vi "CMI Sync V3 Set Channel 1 Division Factor by Desired Freq.vi"(8 "error in":errorcluster, 9 "explicit ref freq [Hz] (0: auto estimate)":dbl, 10 "target output freq [Hz]":dbl=1000.0, 11 "session in":T1={"VISA"="", "baud rate [bd/s]"=115200, "source"=enum."Auto", "hv range"=enum."1kV", "fsrc is fixed"=FALSE, "fsrc [Hz]"=10000000.0, "freq integ [s]"=1.0, "freq filter"=5, "trig level"=enum."TTL 5V", "chn1 mode"=enum."Source divider", "chn1 level"=enum."Positive 5V", "chn2 mode"=enum."Source divider", "chn2 level"=enum."Positive 5V", "chn2 div"=1, "chn3 mode"=enum."Chn 1 Active", "chn3 level"=enum."Positive 5V", "chn1 div entry"=enum."Calculate nearest divisor from measured fx", "chn1 dev limit [%]"=1.0, "chn1 check dev"=FALSE} {"chn2 div" min=1 max=100000000 step=1; "fsrc [Hz]" format="%_8p"}) -> (0 "error out":errorcluster, 1 "divisor":i32, 2 "output freq [Hz]":dbl, 3 "session out":T1={"VISA"="", "baud rate [bd/s]"=115200, "source"=enum."Auto", "hv range"=enum."1kV", "fsrc is fixed"=FALSE, "fsrc [Hz]"=10000000.0, "freq integ [s]"=1.0, "freq filter"=5, "trig level"=enum."TTL 5V", "chn1 mode"=enum."Source divider", "chn1 level"=enum."Positive 5V", "chn2 mode"=enum."Source divider", "chn2 level"=enum."Positive 5V", "chn2 div"=1, "chn3 mode"=enum."Chn 1 Active", "chn3 level"=enum."Positive 5V", "chn1 div entry"=enum."Calculate nearest divisor from measured fx", "chn1 dev limit [%]"=1.0, "chn1 check dev"=FALSE} {"chn2 div" min=1 max=100000000 step=1; "fsrc [Hz]" format="%_8p"})   [LabVIEW 2020, in "AWG.lvlib" / "CMI Sync Unit V3.lvlib"]
doc: "Sets nearest divisor for channel 1 in direct division mode by entering desired frequency and measured source frequency. Returns actual divisor and output frequency."
uses:
  CMI Sync Unit V3.lvlib
  CMI Sync V3 session.ctl
  CMI Sync V3 Reference Clock Source.ctl
  CMI Sync V3 HV input Range.ctl
  CMI Sync V3 Trigger Input Level.ctl
  CMI Sync V3 Channel 1 Mode.ctl
  CMI Sync V3 Channel Output Levels.ctl
  CMI Sync V3 Channel 2 Mode.ctl
  CMI Sync V3 Channel 3 Mode.ctl
  CMI Sync V3 Channel 1 Divisor Entry Mode.ctl
  <vilib>/Utility/error.llb/Error Cluster From Error Code.vi
  <vilib>/ErrorRing/Error Ring.xnode
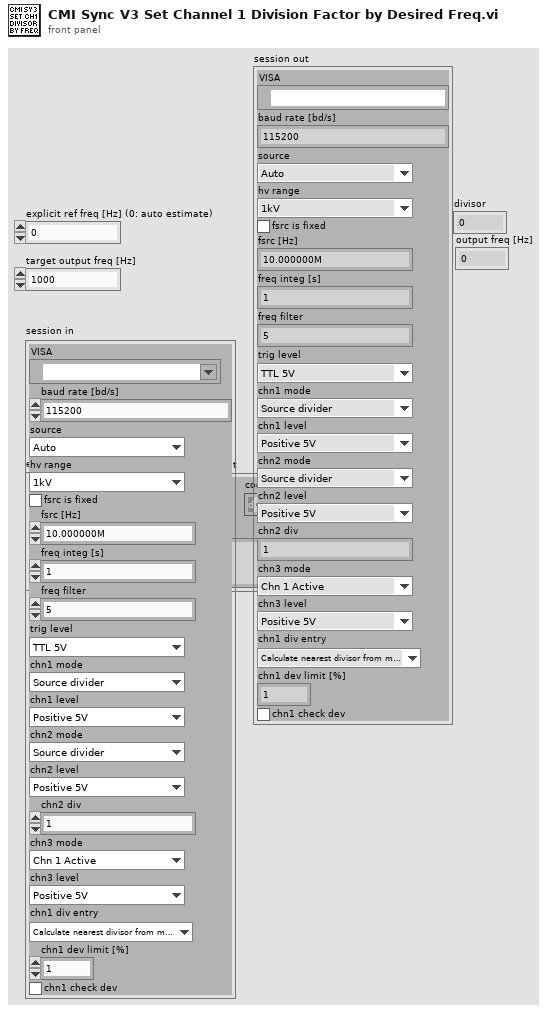
[diagram p1: front panel]
types:
  T1 = typedef "AWG.lvlib/CMI Sync Unit V3.lvlib/CMI Sync V3 session.ctl" = cluster{"VISA":refnum<visa-resource-name>, "baud rate [bd/s]":i32, "source":T2, "hv range":T3, "fsrc is fixed":bool, "fsrc [Hz]":dbl, "freq integ [s]":dbl, "freq filter":i32, "trig level":T4, "chn1 mode":T5, "chn1 level":T6, "chn2 mode":T7, "chn2 level":T6, "chn2 div":i32, "chn3 mode":T8, "chn3 level":T6, "chn1 div entry":T9, "chn1 dev limit [%]":dbl, "chn1 check dev":bool}
  T2 = typedef "AWG.lvlib/CMI Sync Unit V3.lvlib/CMI Sync V3 Reference Clock Source.ctl" = enum16{"Auto", "Internal", "Logic", "Sine", "HV"}
  T3 = typedef "AWG.lvlib/CMI Sync Unit V3.lvlib/CMI Sync V3 HV input Range.ctl" = enum16{"10V", "60V", "250V", "1kV"}
  T4 = typedef "AWG.lvlib/CMI Sync Unit V3.lvlib/CMI Sync V3 Trigger Input Level.ctl" = enum16{"LVCMOS 3V3", "TTL 5V"}
  T5 = typedef "AWG.lvlib/CMI Sync Unit V3.lvlib/CMI Sync V3 Channel 1 Mode.ctl" = enum16{"Source divider", "DDS absolute", "DDS ratio", "DDS ratio M/N"}
  T6 = typedef "AWG.lvlib/CMI Sync Unit V3.lvlib/CMI Sync V3 Channel Output Levels.ctl" = enum16{"Positive 3V3", "Negative 3V3", "Positive 5V", "Negative 5V"}
  T7 = typedef "AWG.lvlib/CMI Sync Unit V3.lvlib/CMI Sync V3 Channel 2 Mode.ctl" = enum16{"Source divider", "Chn 1 divide"}
  T8 = typedef "AWG.lvlib/CMI Sync Unit V3.lvlib/CMI Sync V3 Channel 3 Mode.ctl" = enum16{"Chn 1 Active", "Chn 2 Active", "Chn 1 Trigger", "Chn 2 Trigger", "Gate", "PPS", "10MHz"}
  T9 = typedef "AWG.lvlib/CMI Sync Unit V3.lvlib/CMI Sync V3 Channel 1 Divisor Entry Mode.ctl" = enum16{"Set divisor directly", "Calculate nearest divisor from measured fx"}
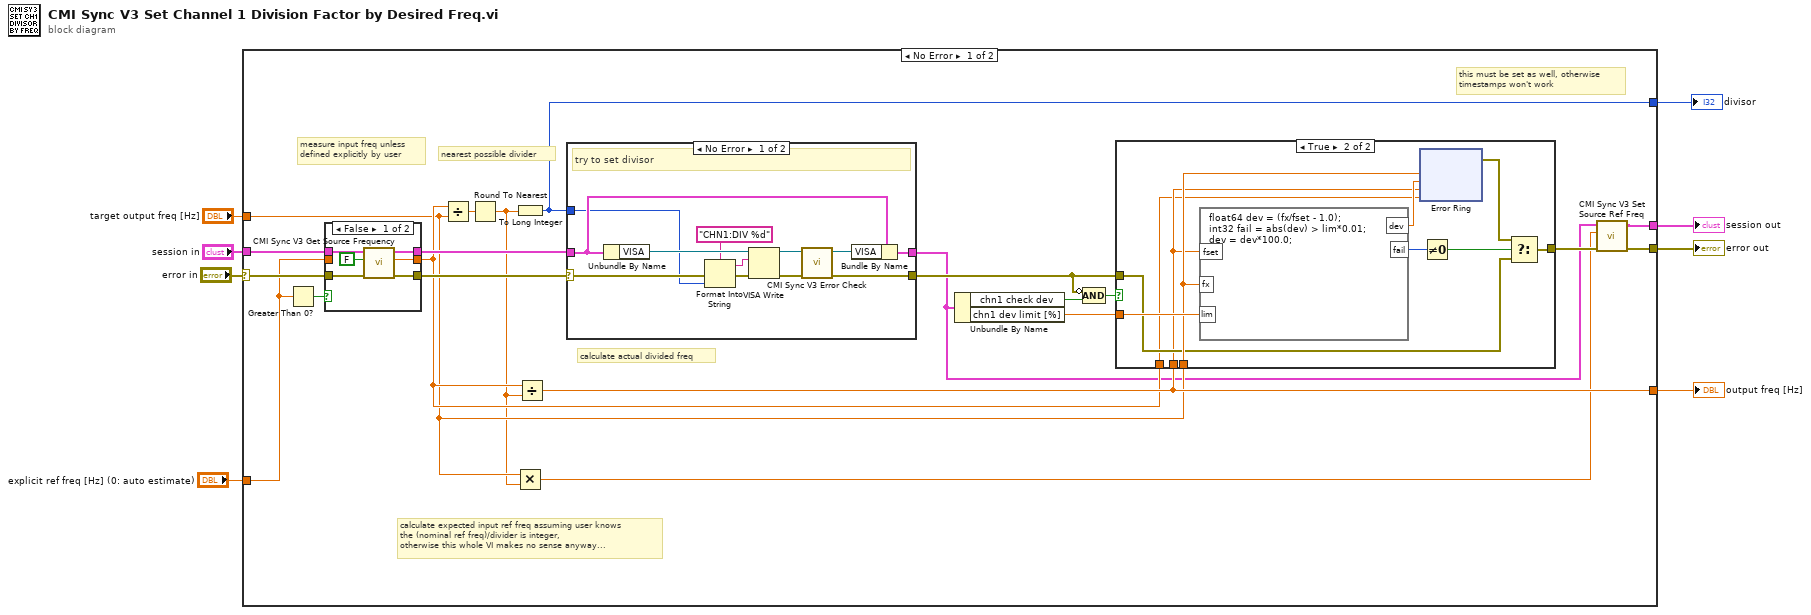
[diagram p0: block diagram]
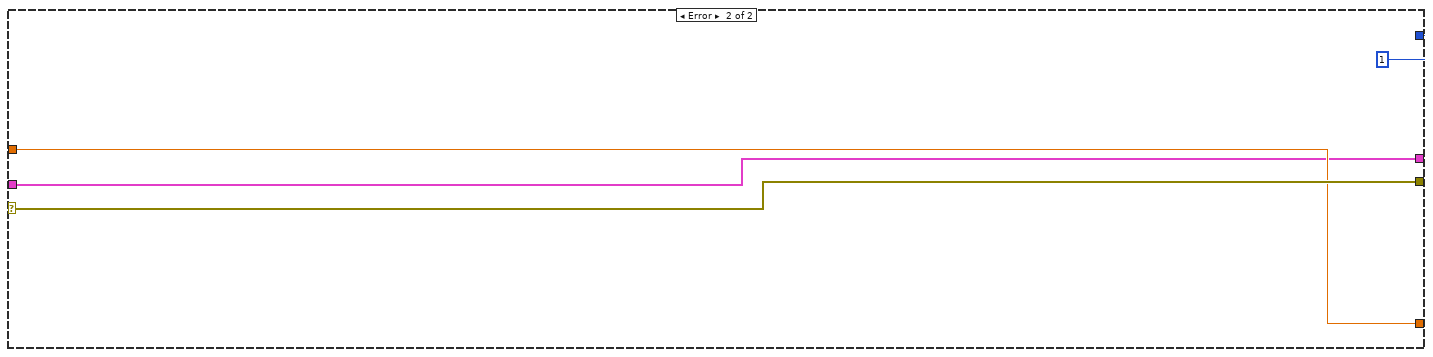
[diagram p5: hidden frame]
diagram:
  n1 = case shown="No Error" "error in" {
    selector: "error in" -> [w29 w77]
    tunnel: "session in" -> [w18 w74]
    tunnel: "target output freq [Hz]" -> [w17 w76]
    tunnel: [w25 1] -> w5
    tunnel: [w20 w76] -> w4
    tunnel: [w13 w77] -> w3
    tunnel: [w12 w74] -> w2
    tunnel: "explicit ref freq [Hz] (0: auto estimate)" -> [w10 _]
    frame No Error {
      # "measure input freq unless\ndefined explicitly by user"
      # "this must be set as well, otherwise\ntimestamps won't work"
      # "calculate expected input ref freq assuming user knows\nthe (nominal ref freq)/divider is integer, \notherwise this whole VI makes no sense anyway..."
      # "calculate actual divided freq"
      # "nearest possible divider"
      n2 = Greater Than 0?(x=w10) -> (x > 0?=w11:bool)
      n3 = case shown="False" w11 {
        tunnel: w29 -> [w34 w38]
        tunnel: [w33 w38] -> w27
        tunnel: [w32 w37] -> w26
        tunnel: [w31 w36] -> w19
        tunnel: w18 -> [w30 w37]
        tunnel: w10 -> [_ w36]
        frame False {
          n4 = call "CMI Sync V3 Get Source Frequency.vi"("error in"=w34, "Wait for update before? (false)"=FALSE, "session in"=w30) -> ("error out"=w33:errorcluster, "source frequency [Hz]"=w31:dbl, "session out"=w32:T1)  [unwired: 6 in]
        }
        frame True {
        }
      }
      n5 = Divide(x=w19, y=w17) -> (x/y=w28:dbl)
      n6 = Round To Nearest(number=w28) -> (nearest integer value=w16:dbl)
      n7 = To Long Integer(number=w16) -> (32bit integer=w25:i32)
      n8 = Multiply(x=w17, y=w16) -> (x*y=w9:dbl)
      n9 = Divide(x=w19, y=w16) -> (x/y=w20:dbl)
      n10 = case shown="No Error" w27 {
        selector: w27 -> [w64 w73]
        tunnel: w26 -> [w71 w72]
        tunnel: [w70 w72] -> w14
        tunnel: [w65 w73] -> w22
        tunnel: w25 -> [w60 _]
        frame No Error {
          # "try to set divisor"
          n11 = Unbundle By Name(w71) -> ("VISA"=w69:refnum<visa-resource-name>)
          n12 = Format Into String(format string="CHN1:DIV %d", error in=w64, w60) -> (resulting string=w62:string, error out=w63:errorcluster)  [unwired: 1 in]
          n13 = VISA Write(VISA resource name=w69, write buffer=w62, error in (no error)=w63) -> (VISA resource name out=w67:refnum<visa-resource-name>, error out=w68:errorcluster)  [unwired: 1 out]
          n14 = call "CMI Sync V3 Error Check.vi"("error in"=w68, "VISA in"=w67) -> ("error out"=w65:errorcluster, "VISA out"=w66:refnum<visa-resource-name>)  [unwired: 7 in, 1 out]
          n15 = Bundle By Name(cluster=w71, "VISA"=w66) -> (w70:T1)
        }
        frame Error {
        }
      }
      n16 = Unbundle By Name(w14) -> ("chn1 check dev"=w24:bool, "chn1 dev limit [%]"=w21:dbl)
      n17 = Compound Arithmetic op=AND(invert w22, w24) -> (w23:bool)
      n18 = case shown="True" w23 {
        tunnel: w22 -> [w39 w44]
        tunnel: w21 -> [_ w49]
        tunnel: w17 -> [_ w46]
        tunnel: w20 -> [_ w41]
        tunnel: w19 -> [_ w40]
        tunnel: [w39 w43] -> w15
        frame False {
        }
        frame True {
          n19 = formula code="float64 dev = (fx/fset - 1.0);\nint32 fail = abs(dev) > lim*0.01;\ndev = dev*100.0;"("fset"=w41, "fx"=w46, "lim"=w49) -> ("fail"=w48:i32, "dev"=w42:dbl)
          n20 = xnode "Error Ring"("parameter 0"=w46, "parameter 1"=w42, "parameter 2"=w41, "parameter 3"=w40) -> ("error out"=w45:errorcluster)
          n21 = Not Equal To 0?(x=w48) -> (x != 0?=w47:bool)
          n22 = Select(t=w45, s=w47, f=w44) -> (s? t:f=w43:errorcluster)
        }
      }
      n23 = call "CMI Sync V3 Set Source Ref Freq.vi"("error in"=w15, "Expected reference frequency [Hz]"=w9, "session in"=w14) -> ("error out"=w13:errorcluster, "session out"=w12:T1)  [unwired: 7 in]
    }
    frame Error {
    }
  }
  "error out" <- w3
  "session out" <- w2
  "divisor" <- w5
  "output freq [Hz]" <- w4
